vi "Configure.vi"(8 "error in":errorcluster, 10 "hw timeout (sec)":dbl=30.0 format="%#_13g") -> (0 "error out":errorcluster, 2 "watchdogID out":u64, 3 "Pound":refnum<class "Pound.lvclass">)   [LabVIEW 2017, in "WatchdogProcess.lvlib"]
doc: "Specifies the length of the hardware timeout period that triggers a recovery procedure."
uses:
  <vilib>/addons/WatchdogProcess/WatchdogProcess.lvlib
  <vilib>/NI/Software Watchdog/Pound/Pound.lvclass
  <vilib>/RTwatchdog.llb/Watchdog expiration actions.ctl
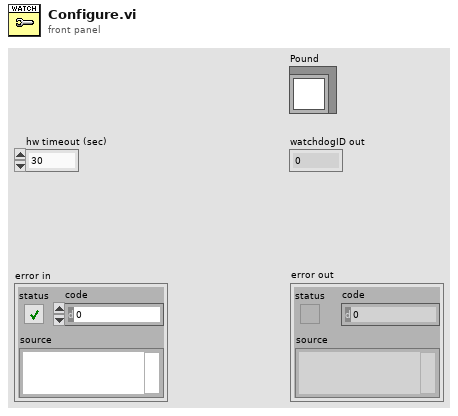
[diagram p1: front panel]
types:
  T1 = typedef "Watchdog expiration actions.ctl" = cluster{"reset system":bool, "restart LabVIEW Runtime":bool, "occurrence":bool, "trigger protocol":enum16{"active high", "active low", "open collector"}, "trigger line":enum16{"none", "line 0", "line 1", "line 2", "line 3", "line 4", "line 5", "line 6", "line 7", "SMB line 0"}, "disable watchdog on VI exit":bool}
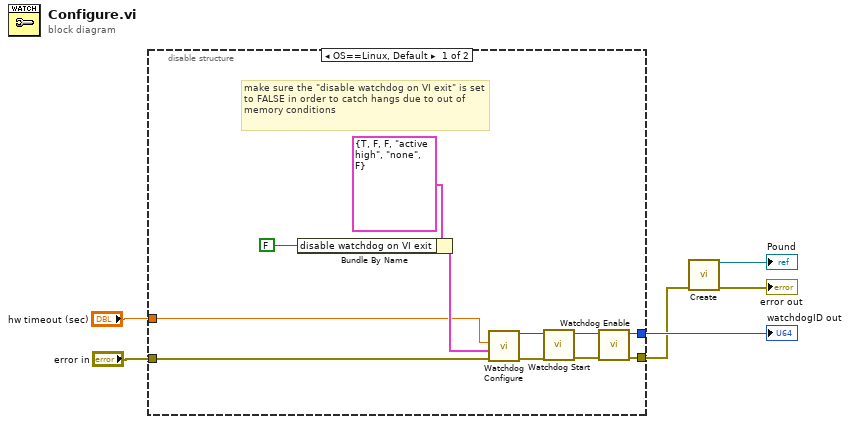
[diagram p0: block diagram]
diagram:
  n1 = disable-structure shown="OS==Linux, Default" {
    disable-tunnel: [w17 _] -> w5
    disable-tunnel: [w16 w18] -> w4
    disable-tunnel: "error in" -> [w12 w18]
    disable-tunnel: "hw timeout (sec)" -> [w7 _]
    frame condition #0 (active) {
      # "make sure the \"disable watchdog on VI exit\" is set to FALSE in order to catch hangs due to out of memory conditions"
      n2 = Bundle By Name(cluster=T1 {"reset system"=TRUE, "restart LabVIEW Runtime"=FALSE, "occurrence"=FALSE, "trigger protocol"=enum."active high", "trigger line"=enum."none", "disable watchdog on VI exit"=FALSE} ("expiration actions"), "disable watchdog on VI exit"=FALSE) -> (w14:T1)
      n3 = call <vilib>:"Watchdog Configure.vi"("error in (no error)"=w12, "expiration actions"=w14, "timeout (1 sec)"=w7) -> ("error out"=w9:errorcluster, "watchdogID"=w8:u64)  [unwired: 1 in, 2 out]
      n4 = call <vilib>:"Watchdog Start.vi"("error in (no error)"=w9, "watchdogID in"=w8) -> ("error out"=w10:errorcluster, "watchdogID out"=w11:u64)  [unwired: 4 in]
      n5 = call <vilib>:"Watchdog Enable.vi"("error in (no error)"=w10, "watchdogID in"=w11) -> ("error out"=w16:errorcluster, "watchdogID out"=w17:u64)  [unwired: 4 in]
    }
    frame condition #1 {
    }
  }
  "watchdogID out" <- w5
  n6 = call <vilib>:"Create.vi"("error in (no error)"=w4) -> ("error out"=→"error out":errorcluster, "Pound"=→"Pound":refnum<class "Pound.lvclass">)  [unwired: 9 in]
